vi "DAQList_GetMeasureValue.vi"(8 "error in (no error)":errorcluster caption="错误输入（无错误）", 11 "Channel Tag[]":string[](array[string])) -> (0 "error out":errorcluster caption="错误输出", 3 "Channels Value":string[](array[string]))   [LabVIEW 2016]
uses:
  <vilib>/Analysis/NI_AALBase.lvlib
  <vilib>/Analysis/baseanly.llb/Mean (DBL).vi
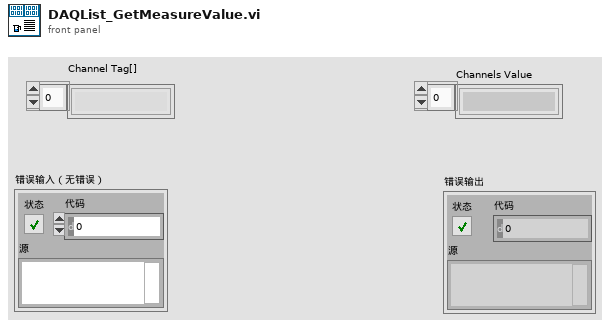
[diagram p1: front panel]
types:
  T1 = cluster{"Queue Name":string, "DAQ Channels":string[], "Queue Type":string}[]
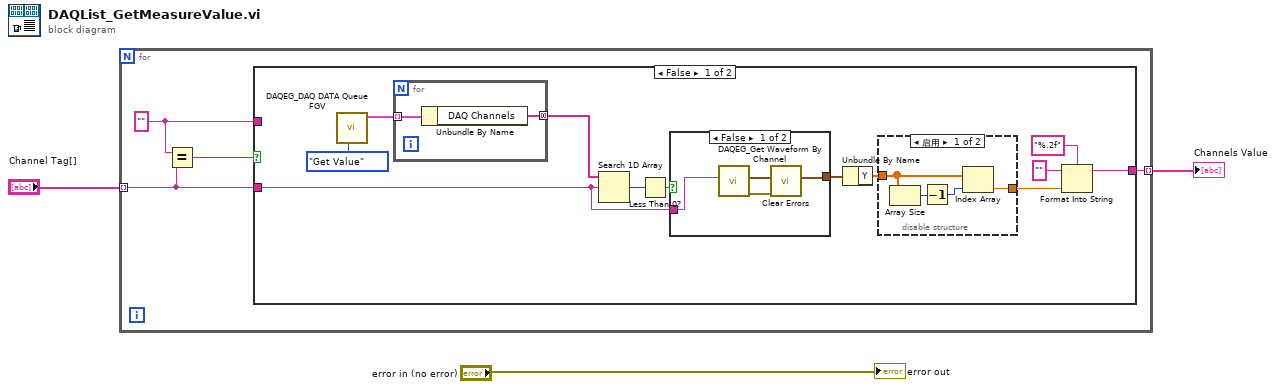
[diagram p0: block diagram]
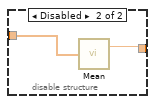
[diagram p2: hidden frame]
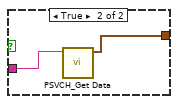
[diagram p3: hidden frame]
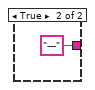
[diagram p4: hidden frame]
diagram:
  n1 = for {
    tunnel: "Channel Tag[]" -> [w6] mode=indexing
    tunnel: [w7] -> w3 mode=indexing
    w4 = "" ("x")
    n2 = Equal?(x=w4, y=w6) -> (x = y?=w5:bool)
    n3 = case shown="False" w5 {
      tunnel: w6 -> [w14 _]
      tunnel: [w8 "---"] -> w7
      tunnel: w4 -> [_ _]
      frame False {
        n4 = call "DAQEG_DAQ DATA Queue FGV.vi"("Command"=enum16{"Initialize", "Get Value", "Set Value"}."Get Value") -> ("DAQ DATA Out"=w18:T1)  [unwired: 9 in, 1 out]
        n5 = for {
          tunnel: w18 -> [w27] mode=indexing
          tunnel: [w26] -> w19 mode=concatenating
          n6 = Unbundle By Name(w27) -> ("DAQ Channels"=w26:string[])
        }
        n7 = Search 1D Array(1D array=w19, element=w14) -> (index of element=w15:i32)  [unwired: 1 in]
        n8 = Less Than 0?(x=w15) -> (x < 0?=w16:bool)
        n9 = case shown="False" w16 {
          tunnel: w14 -> [w30 w32]
          tunnel: [w29 w31] -> w13
          frame False {
            n10 = call "DAQEG_Get Waveform By Channel.vi"("DAQ Channel"=w30) -> ("error out"=w28:errorcluster, "waveform"=w29:waveform(dbl))  [unwired: 9 in]
            n11 = call <vilib>:"Clear Errors.vi"("error in (no error)"=w28) -> ()  [unwired: 5 in, 2 out]
          }
          frame True {
            n12 = call "PSVCH_Get Data.vi"("ChlName"=w32) -> ("Data"=w31:waveform(dbl))  [unwired: 8 in, 2 out]
          }
        }
        n13 = Unbundle By Name(w13) -> ("Y"=w12:dbl[])
        n14 = disable-structure shown="启用" {
          disable-tunnel: w12 -> [w21 w24]
          disable-tunnel: [w20 w25] -> w9
          frame Enabled {
            n15 = Array Size(array=w21) -> (size(s)=w23:i32)
            n16 = Decrement(x=w23) -> (x-1=w22:i32)
            n17 = Index Array(array=w21, index=w22) -> (element=w20:dbl)
          }
          frame Disabled {
            n18 = call-poly <vilib>:"Mean.vi"("X"=w24) -> ("mean"=w25:dbl)  [unwired: 1 out]
          }
        }
        n19 = Format Into String(format string="%.2f", initial string="", w9) -> (resulting string=w8:string)  [unwired: 1 in, 1 out]
      }
      frame True {
      }
    }
  }
  "Channels Value" <- w3
  "error out" <- "error in (no error)"
